vi "Close Pop-Up.vi"(8 "error in":errorcluster) -> (0 "error out":errorcluster)   [LabVIEW 2021, in "Pop-Up.lvlib" / "Popup.lvclass"]
doc: "This VI can be used to close the pop-up early before the user has finished interacting or it has completed its action.\n\nFor example, a timeout dialog can be implemented with an approximate time for an action, but could be closed early if the action finishes before the dialog is complete.\n\n<b>Code Developed By:</b> +\nDaniel Coons +\nhttps://github.com/danielcoons/tsc-pop-up"
uses:
  Popup.lvclass
  Popup.lvclass/Popup.ctl
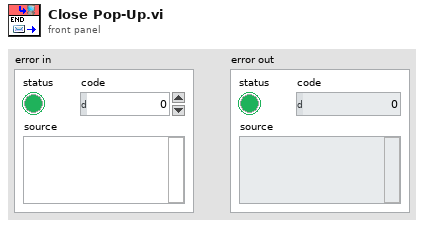
[diagram p1: front panel]
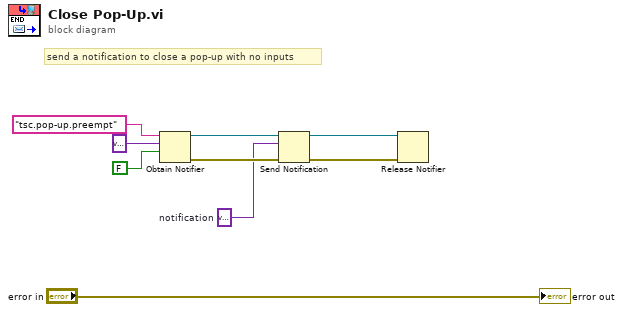
[diagram p0: block diagram]
diagram:
  w2 = variant  # notification
  # "send a notification to close a pop-up with no inputs"
  n1 = Obtain Notifier(name (unnamed)="tsc.pop-up.preempt", notification data type=variant, create if not found? (T)=FALSE) -> (notifier out=w4:refnum<notifier>, error out=w8:errorcluster)  [unwired: 1 in, 1 out]
  n2 = Send Notification(notification=w2, notifier=w4, error in (no error)=w8) -> (notifier out=w3:refnum<notifier>, error out=w7:errorcluster)
  n3 = Release Notifier(notifier=w3, error in (no error)=w7) -> ()  [unwired: 1 in, 3 out]
  "error out" <- "error in"
